vi "NeoProducer.vi"(8 "Error In":errorcluster) -> (0 "Error Out":errorcluster)   [LabVIEW 2014]
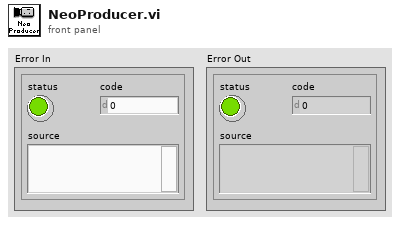
[diagram p1: front panel]
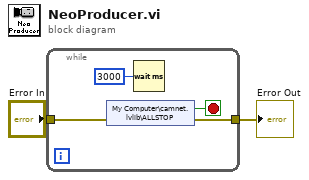
[diagram p0: block diagram]
diagram:
  n1 = while {
    tunnel: "Error In" -> [w5]
    tunnel: [w4] -> w1
    stop <- w6 stop-if-true
    n2 = shared-variable "My Computer\\camnet.lvlib\\ALLSTOP"(error in=w5) -> (w6:bool, error out=w4:errorcluster)
    n3 = Wait (ms)(milliseconds to wait=u32 3000) -> ()  [unwired: 1 out]
  }
  "Error Out" <- w1
